vi "Installer Post-Install Action.vi"   [LabVIEW 2015]
uses:
  <vilib>/Utility/sysdir.llb/System Directory Type.ctl
types:
  T1 = typedef "System Directory Type.ctl" = i32
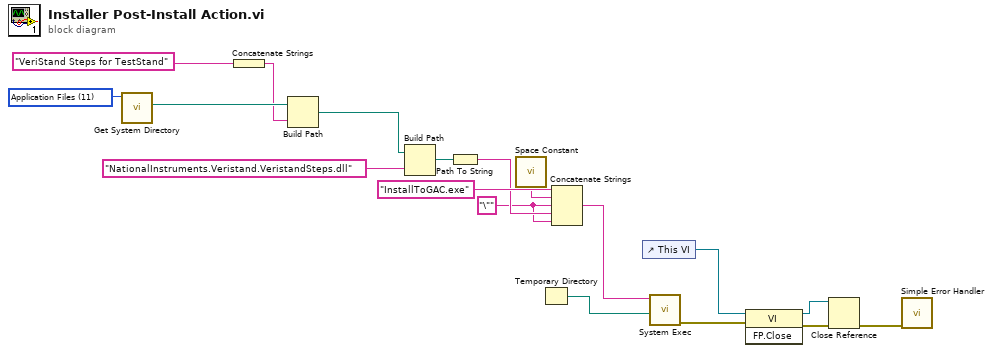
[diagram p0: block diagram]
diagram:
  w3 = T1 11 items=["User Home"=0, "User Desktop"=1, "User Documents"=2, "User Application Data"=3, "User Preferences"=4, "User Temporary"=5, "Public Documents"=6, "Public Application Data"=7, "Public Preferences"=8, "Public Cache"=13, "System Core Libraries"=9, "System Installed Libraries"=10, "Application Files"=11, "Boot Volume Root"=12] ("system directory type")
  w8 = "\"" ("string")
  n1 = call <vilib>:"Get System Directory.vi"("system directory type"=w3) -> ("system directory"=w4:path)  [unwired: 10 in]
  n2 = Concatenate Strings("VeriStand Steps for TestStand") -> (w1:string)
  n3 = Build Path(base path=w4, name or relative path=w1) -> (appended path=w2:path)
  n4 = Build Path(base path=w2, name or relative path="NationalInstruments.Veristand.VeristandSteps.dll" ("command line")) -> (appended path=w15:path)
  n5 = Path To String(path=w15) -> (string=w9:string)
  n6 = call <vilib>:"Space Constant.vi"() -> ("String"=w16:string)
  n7 = Temporary Directory() -> (w6:path)
  n8 = Concatenate Strings("InstallToGAC.exe" ("command line"), w16, w8, w9, w8) -> (w7:string)
  n9 = control-ref of="This VI"() -> (w14:refnum<vi>)
  n10 = call <vilib>:"System Exec.vi"("working directory"=w6, "command line"=w7) -> ("error out"=w10:errorcluster)  [unwired: 6 in, 3 out]
  n11 = invoke class="VI" method="FP.Close"(reference=w14, error in=w10) -> (reference out=w11:refnum<vi>, error out=w12:errorcluster)  [unwired: 1 in, 1 out]
  n12 = Close Reference(reference=w11, error in (no error)=w12) -> (error out=w13:errorcluster)
  n13 = call <vilib>:"Simple Error Handler.vi"("error in (no error)"=w13) -> ()  [unwired: 4 in, 5 out]
